vi "Do.vi"(8 "error in (no error)":errorcluster, 9 "Events":refnum<class "Events.lvclass">, 10 "Message Loop Data in":T1, 11 "IInternalRequest in":refnum<class "UnregisteredHandler.lvclass">) -> (0 "error out":errorcluster, 2 "Message Loop Data out":T1, 3 "IInternalRequest out":refnum<class "UnregisteredHandler.lvclass">)   [LabVIEW 2020, in "wamplv.lvlib" / "UnregisteredHandler.lvclass"]
uses:
  UnregisteredHandler.lvclass
  UnregisteredHandler.lvclass/UnregisteredHandler.ctl
  SerialisedMessages/JSONMessage/WampMessage JSON.lvclass
  Error/ErrorHandler JSON/ErrorHandler JSON.lvclass
  Unregister/Unregister JSON/Unregister JSON.lvclass
  WAMP Client/Private/TypeDef/Success or error (JSON).ctl
  wamplv.lvlib
  WAMP Client/API/TypeDefs/Error or abort detail (JSON).ctl
  <vilib>/ErrorRing/Error Ring.xnode
  <vilib>/Utility/error.llb/Error Cluster From Error Code.vi
  WAMP Client/Private/TypeDef/Publish Requests Map.ctl
  WAMP Client/Private/TypeDef/Endpoint Data.ctl
  Call/ICallRequest/ICallRequest.lvclass
  WAMP Client/Private/TypeDef/CALL Request Map.ctl
  WAMP Client/Private/TypeDef/SUBSCRIBE Requests Map.ctl
  WAMP Client/Private/TypeDef/Subscriptions Map.ctl
  WAMP Client/Private/TypeDef/Unsubscribe Requests Map.ctl
  WAMP Client/Private/TypeDef/Unregister requests map.ctl
  WAMP Client/Private/TypeDef/Message Loop Data.ctl
  Events/EventsParent/Events.lvclass
  Subscribe/ISubscribe/ISubscribe.lvclass
  Publish/IPublish/IPublish.lvclass
  Message loop classes/Subscription details/SubscriptionDetailsParent/SubscriptionDetailsParent.lvclass
  Unsubscribe/IUnsubscribe/IUnsubscribe.lvclass
  Register/IRegister/IRegister.lvclass
  Unregister/IUnregister/IUnregister.lvclass
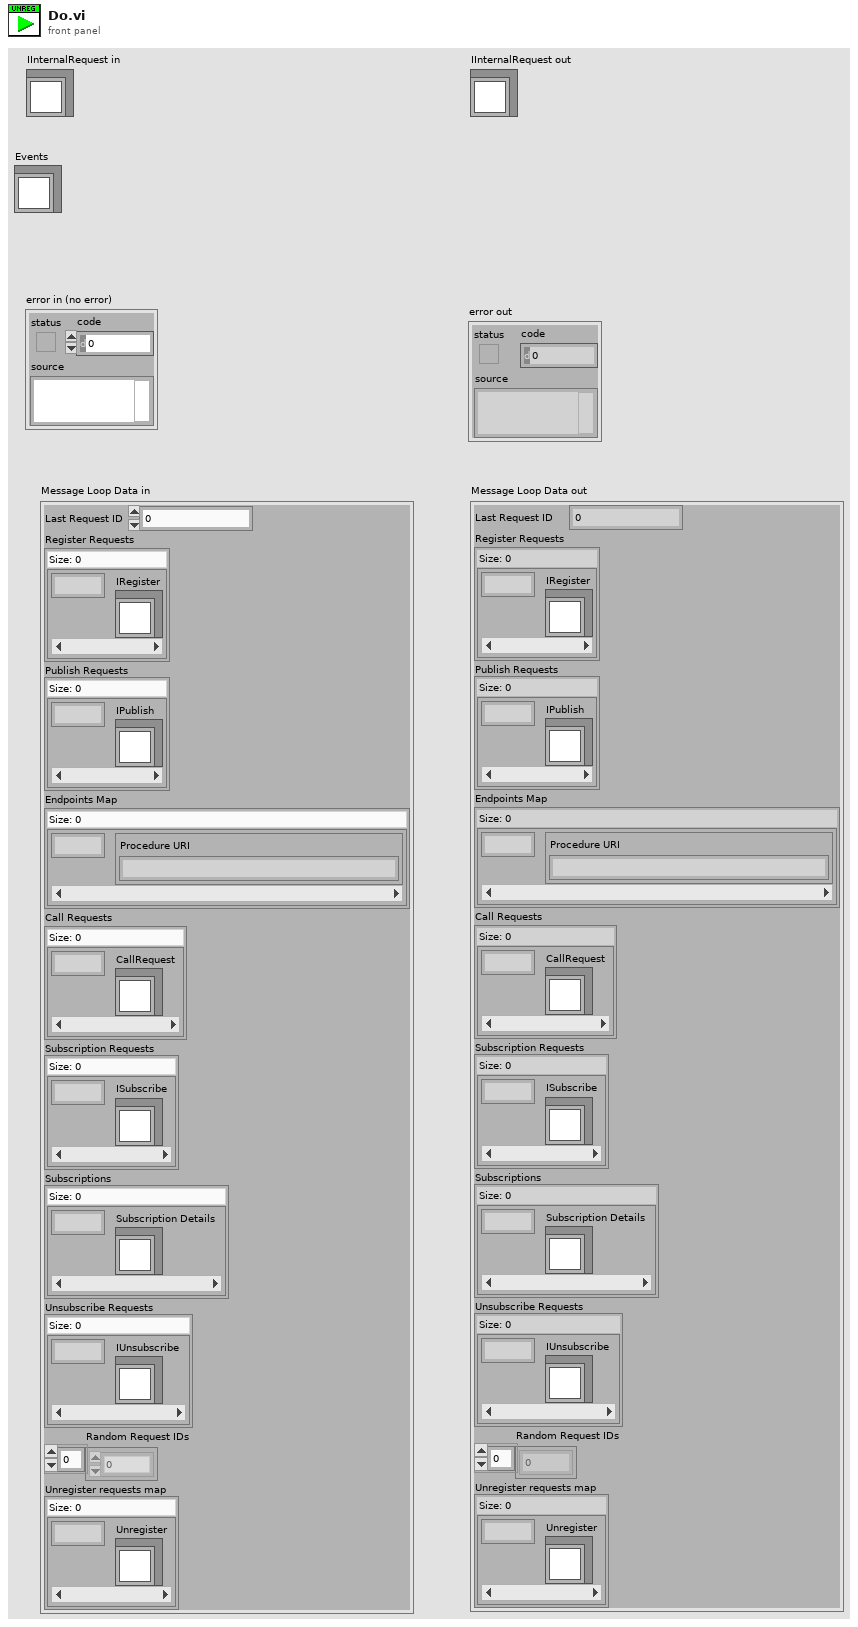
[diagram p1: front panel]
types:
  T1 = typedef "wamplv.lvlib/Message Loop Data.ctl" = cluster{"Last Request ID":u64, "Register Requests":map{u64, refnum<class "IRegister.lvclass">}, "Publish Requests":T2, "Endpoints Map":map{u64, T3}, "Call Requests":T4, "Subscription Requests":T5, "Subscriptions":T6, "Unsubscribe Requests":T7, "Random Request IDs":u64[], "Unregister requests map":T8}
  T2 = typedef "wamplv.lvlib/Publish Requests Map.ctl" = map{u64, refnum<class "IPublish.lvclass">}
  T3 = typedef "wamplv.lvlib/Endpoint Data.ctl" = cluster{"Procedure URI":string}
  T4 = typedef "wamplv.lvlib/CALL Request Map.ctl" = map{u64, refnum<class "ICallRequest.lvclass">}
  T5 = typedef "wamplv.lvlib/SUBSCRIBE Requests Map.ctl" = map{u64, refnum<class "ISubscribe.lvclass">}
  T6 = typedef "wamplv.lvlib/Subscriptions Map.ctl" = map{u64, refnum<class "SubscriptionDetailsParent.lvclass">}
  T7 = typedef "wamplv.lvlib/Unsubscribe Requests Map.ctl" = map{u64, refnum<class "IUnsubscribe.lvclass">}
  T8 = typedef "wamplv.lvlib/Unregister requests map.ctl" = map{u64, refnum<class "IUnregister.lvclass">}
  T9 = typedef "wamplv.lvlib/Success or error (JSON).ctl" = cluster{"Success?":bool, "URI":string, "Error/Abort details (JSON)":T10}
  T10 = typedef "wamplv.lvlib/Error or abort detail (JSON).ctl" = cluster{"URI":string, "Arguments Payload":string, "ArgumentKw Payload":string, "Details":string, "Associated LabVIEW Error":errorcluster}
  T11 = typedef "wamplv.lvlib/WAMP Message Codes.ctl" = enum8{"HELLO", "WELCOME", "CHALLENGE", "AUTHENTICATE", "ABORT", "GOODBYE", "ERROR", "PUBLISH", "PUBLISHED", "SUBSCRIBE", "SUBSCRIBED", "UNSUBSCRIBE", "UNSUBSCRIBED", "EVENT", "CALL", "RESULT", "REGISTER", "REGISTERED", "UNREGISTER", "UNREGISTERED", "INVOCATION", "YIELD"}
  T12 = typedef "wamplv.lvlib/Error (JSON).ctl" = cluster{"Request ID":u64, "Message type that caused error":T11, "Error/Abort details (JSON)":T10}
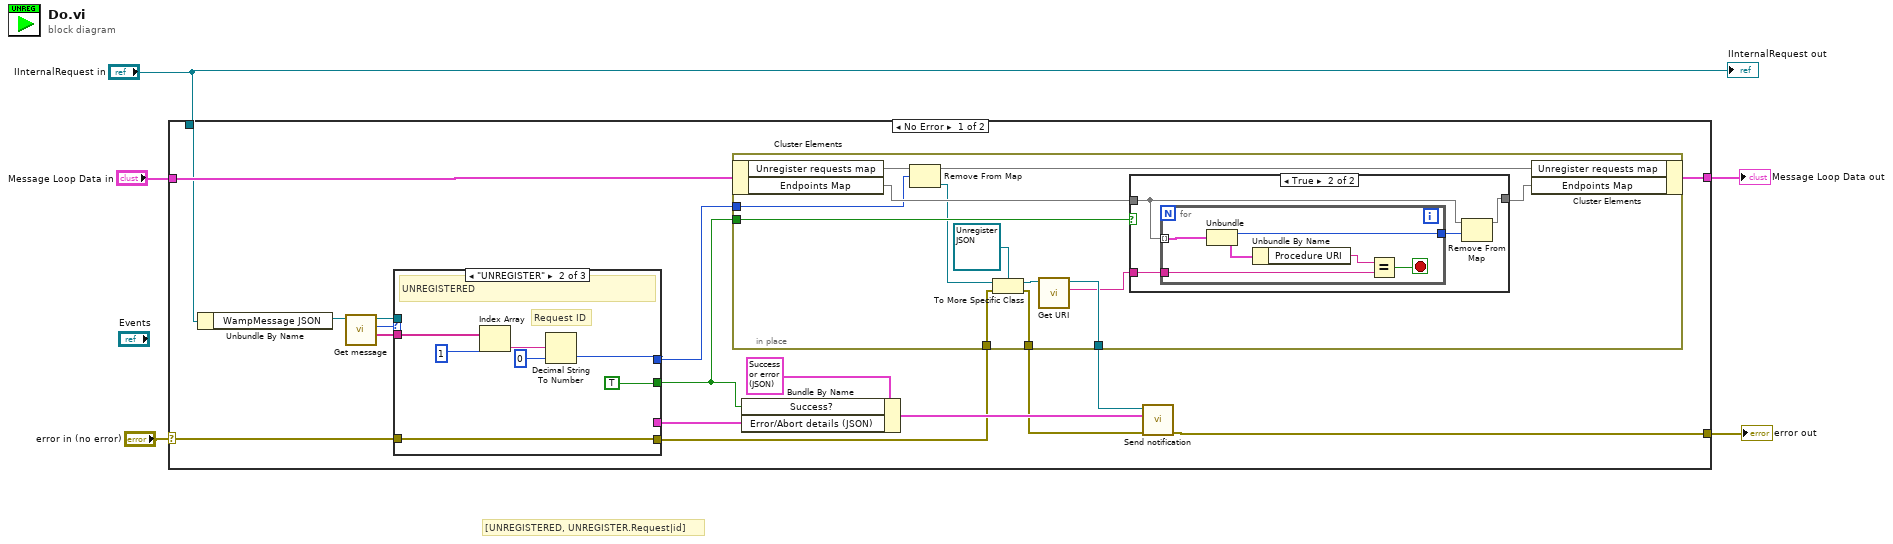
[diagram p0: block diagram]
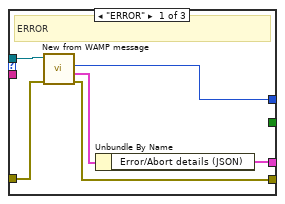
[diagram p3: hidden frame]
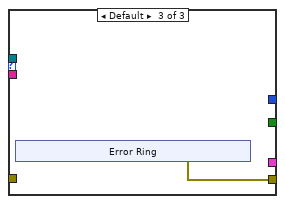
[diagram p4: hidden frame]
diagram:
  # "[UNREGISTERED, UNREGISTER.Request|id]"
  n1 = case shown="No Error" "error in (no error)" {
    selector: "error in (no error)" -> [w19 w65]
    tunnel: "Message Loop Data in" -> [w18 w66]
    tunnel: [w7 w65] -> w3
    tunnel: [w17 w66] -> w2
    tunnel: "IInternalRequest in" -> [w16 _]
    frame No Error {
      n2 = Unbundle By Name(w16) -> ("WampMessage JSON"=w15:refnum<class "WampMessage JSON.lvclass">)
      n3 = call "Get message.vi"("JSONMessage in"=w15) -> ("<JSON>Elements"=w13:string[], "Message Type"=w14:T11, "JSONMessage out"=w12:refnum<class "WampMessage JSON.lvclass">)  [unwired: 8 in]
      n4 = case shown="\"UNREGISTER\"" w14 {
        tunnel: w13 -> [_ w58 _]
        tunnel: [w49 w53 _] -> w20
        tunnel: w19 -> [w52 w57 _]
        tunnel: [w50 w57 w60] -> w6
        tunnel: [w47 _ _] -> w22
        tunnel: [_ TRUE ("Success?") _] -> w11
        tunnel: w12 -> [w51 _ _]
        frame "ERROR" {
          # "ERROR"
          n5 = call "New from WAMP message.vi"("error in (no error)"=w52, "wamplv.lvlib:JSONMessage.lvclass"=w51) -> ("error out"=w50:errorcluster, "Error data (JSON)"=w48:T12, "Request ID"=w49:u64)  [unwired: 6 in, 1 out]
          n6 = Unbundle By Name(w48) -> ("Error/Abort details (JSON)"=w47:T10)
        }
        frame "UNREGISTER" {
          # "Request ID"
          # "UNREGISTERED"
          n7 = Index Array(array=w58, index=1) -> (element=w55:string)
          n8 = Decimal String To Number(string=w55, default (0L)=u64 0) -> (number=w53:u64)  [unwired: 1 in, 1 out]
        }
        frame Default {
          n9 = xnode "Error Ring"() -> ("error out"=w60:errorcluster)
        }
      }
      n10 = in-place {
        in-place-border: w20 -> [w31]
        in-place-border: w11 -> [w30]
        in-place-border: [w26] -> w9
        in-place-border: [w25] -> w8
        in-place-border: w6 -> [w23]
        n11 = in-place-cluster #1(w18) -> ("Unregister requests map"=w35:T8, "Endpoints Map"=w33:map{u64, T3})
        n12 = Remove From Map(10:w31, 11:w35) -> (1:w28:refnum<class "IUnregister.lvclass">, 3:w34:T8)  [unwired: 1 out]
        n13 = To More Specific Class(target class=refnum<class "Unregister JSON.lvclass"> refnum ("wamplv.lvlib:Unregister JSON.lvclass"), reference=w28, error in=w23) -> (specific class reference=w27:refnum<class "Unregister JSON.lvclass">, error out=w25:errorcluster)
        n14 = call-dynamic "Get URI.vi"("Unregister JSON in"=w27) -> ("URL"=w24:string, "Unregister JSON out"=w26:refnum<class "Unregister JSON.lvclass">)  [unwired: 9 in]
        n15 = case shown="True" w30 {
          tunnel: w24 -> [_ w40]
          tunnel: w33 -> [w36 w38]
          tunnel: [w36 w37] -> w32
          frame False {
          }
          frame True {
            n16 = for {
              tunnel: [w44] -> w39
              tunnel: w38 -> [w42] mode=indexing
              tunnel: w40 -> [w41]
              stop <- w45 stop-if-true
              n17 = Unbundle(w42) -> ("key"=w44:u64, "Endpoint Data"=w46:T3)
              n18 = Unbundle By Name(w46) -> ("Procedure URI"=w43:string)
              n19 = Equal?(x=w43, y=w41) -> (x = y?=w45:bool)
            }
            n20 = Remove From Map(10:w39, 11:w38) -> (3:w37:map{u64, T3})  [unwired: 2 out]
          }
        }
        n21 = in-place-cluster #1("Unregister requests map"=w34, "Endpoints Map"=w32) -> (w17:T1)
      }
      n22 = Bundle By Name(cluster=T9 {"Success?"=FALSE, "URI"="", "Error/Abort details (JSON)"={"URI"="", "Arguments Payload"="", "ArgumentKw Payload"="{}", "Details"="{}", "Associated LabVIEW Error"={"status"=FALSE, "code"=0, "source"=""}}} ("Sucess or error"), "Success?"=w11, "Error/Abort details (JSON)"=w22) -> (w10:T9)
      n23 = call "Send notification.vi"("error in (no error)"=w8, "Unregister result"=w10, "Unregister JSON in"=w9) -> ("error out"=w7:errorcluster)  [unwired: 7 in, 1 out]
    }
    frame Error {
    }
  }
  "error out" <- w3
  "Message Loop Data out" <- w2
  "IInternalRequest out" <- "IInternalRequest in"
